vi "UploadFiles.vi"(7 "Code":string, 8 "error in (no error)":errorcluster, 9 "Python in":T1, 10 "name":string, 11 "Console":refnum<vi>) -> (0 "error out":errorcluster, 2 "Console out":string, 3 "Python out":T1)   [LabVIEW 2022 SP3]
uses:
  PythonCtrl.ctl
  Processors.ctl
panel:
  # "https://github.com/ceeoinnovations/Arduino-cli-setup"
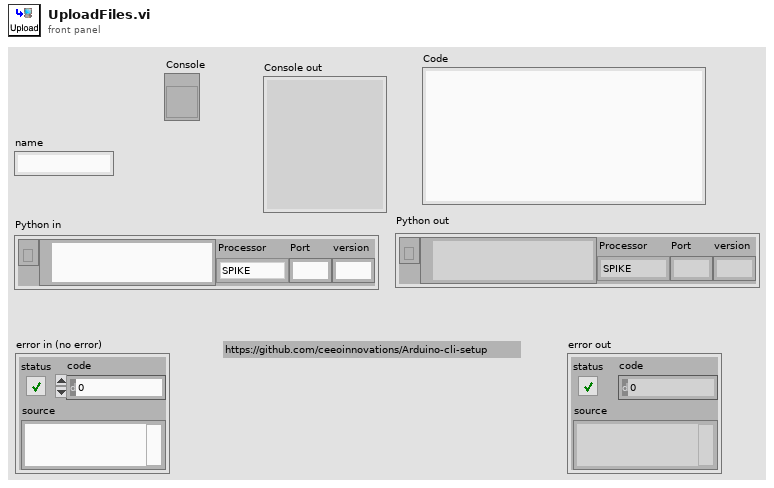
[diagram p1: front panel]
types:
  T1 = typedef "PythonCtrl.ctl" = cluster{"session":refnum<k35>, "PyPath":path, "Processor":T2, "Port":string, "version":string}
  T2 = typedef "Processors.ctl" = enum16{"SPIKE", "Pi", "Pi_ssh", "OpenMV", "Dunio"}
  T3 = typedef "ArduinoCtrl.ctl" = cluster{"CLI directory":path, "Connection":string[], "Code Directory":path}
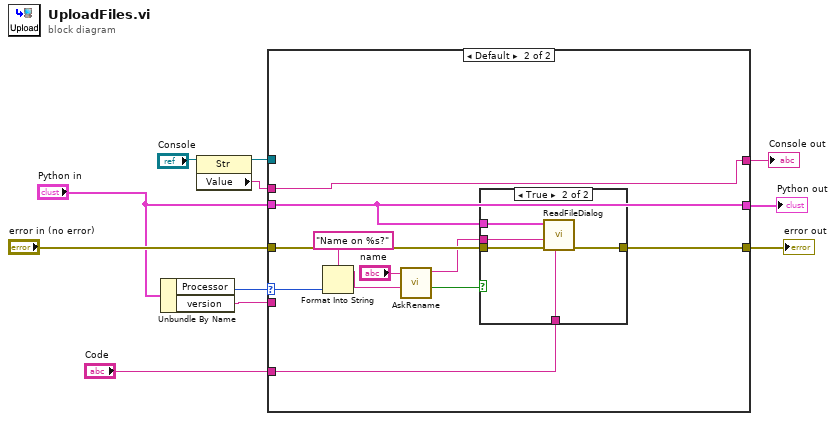
[diagram p0: block diagram]
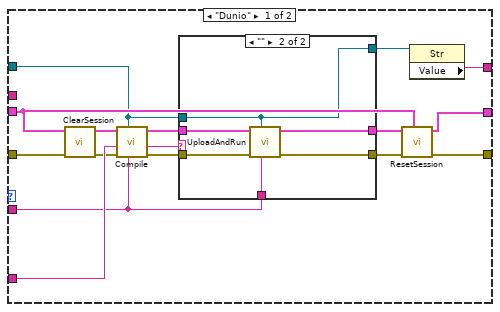
[diagram p2: hidden frame]
diagram:
  n1 = Unbundle By Name("Python in") -> ("Processor"=w7:T2, "version"=w1:string)
  n2 = property class="Str"(reference="Console") -> (reference out=w5:refnum<vi>, "Value"=w4:string)  [unwired: 1 in, 1 out]
  n3 = case shown="Default" w7 {
    selector: w7 -> [_ w39]
    tunnel: "Code" -> [w26 w47]
    tunnel: "error in (no error)" -> [w23 w46]
    tunnel: [w24 w42] -> w9
    tunnel: "Python in" -> [w20 w37]
    tunnel: w5 -> [w15 _]
    tunnel: w4 -> [_ w38]
    tunnel: [w13 w38] -> w3
    tunnel: [w17 w37] -> w2
    tunnel: w1 -> [w12 _]
    frame "Dunio" {
      n4 = call "ClearSession.vi"("error in (no error)"=w23, "Python in"=w20) -> ("error out"=w21:errorcluster, "Arduino"=w22:T3)  [unwired: 8 in]
      n5 = call "Compile.vi"("Python version"=w12, "Console"=w15, "error in"=w21, "Code"=w26, "Arduino in"=w22) -> ("error out"=w25:errorcluster, "standard error"=w16:string, "Arduino out"=w27:T3)  [unwired: 3 in, 1 out]
      n6 = case shown="\"\"" w16 {
        tunnel: w27 -> [w29 w36]
        tunnel: w25 -> [w30 w35]
        tunnel: [w29 w34] -> w19
        tunnel: [w30 w33] -> w18
        tunnel: w15 -> [w28 w32]
        tunnel: [w28 w32] -> w14
        tunnel: w12 -> [_ w31]
        frame Default {
        }
        frame "" {
          n7 = call "UploadAndRun.vi"("Python version"=w31, "Console"=w32, "error in"=w35, "Arduino in"=w36) -> ("error out"=w33:errorcluster, "Arduino out"=w34:T3)  [unwired: 4 in, 2 out]
        }
      }
      n8 = call "ResetSession.vi"("Python in"=w20, "error in"=w18, "Arduino in"=w19) -> ("error out"=w24:errorcluster, "Python out"=w17:T1)  [unwired: 7 in]
      n9 = property class="Str"(reference=w14) -> ("Value"=w13:string)  [unwired: 1 in, 2 out]
    }
    frame Default {
      n10 = Format Into String(format string="Name on %s?" ("Prompt"), w39) -> (resulting string=w40:string)  [unwired: 2 in, 1 out]
      n11 = call "AskRename.vi"("Prompt"=w40, "name"="name") -> ("OK?"=w44:bool, "name 2"=w43:string)  [unwired: 8 in]
      n12 = case shown="True" w44 {
        tunnel: w37 -> [_ w53]
        tunnel: w46 -> [w48 w52]
        tunnel: [w48 w51] -> w42
        tunnel: w43 -> [_ w50]
        tunnel: w47 -> [_ w49]
        frame False {
        }
        frame True {
          n13 = call "ReadFileDialog.vi"("File Text"=w49, "error in (no error)"=w52, "File name"=w50, "Python in"=w53) -> ("error out"=w51:errorcluster)  [unwired: 6 in, 1 out]
        }
      }
    }
  }
  "error out" <- w9
  "Console out" <- w3
  "Python out" <- w2
